vi "BU-SearchParamSpace.vi"(9 "Input String":string, 11 "UCF Param":string[][](table)) -> (2 "Req Param":string[](array[string]))   [LabVIEW 2014]
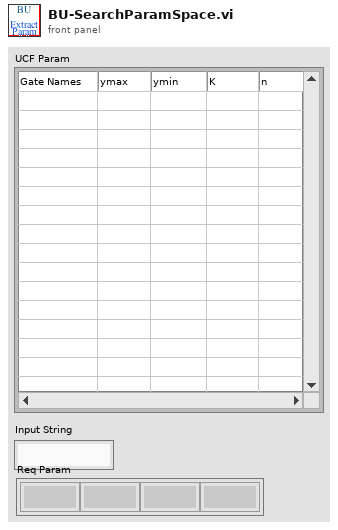
[diagram p1: front panel]
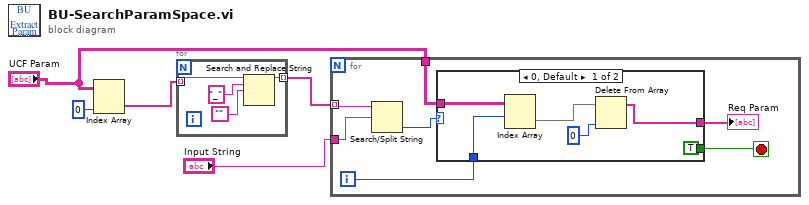
[diagram p0: block diagram]
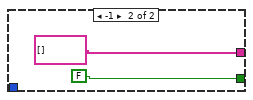
[diagram p2: hidden frame]
diagram:
  n1 = Index Array(array="UCF Param", index (col)=0 ("disabled index (col)")) -> (element=w2:string[])  [unwired: 1 in]
  n2 = for {
    tunnel: w2 -> [w7] mode=indexing
    tunnel: [w6] -> w1 mode=indexing
    n3 = Search and Replace String(input string=w7, search string="_", replace string="") -> (result string=w6:string)  [unwired: 5 in, 3 out]
  }
  n4 = for {
    tunnel: w1 -> [w16] mode=indexing
    tunnel: "Input String" -> [w15]
    tunnel: "UCF Param" -> [w13]
    i -> [w12]
    stop <- w11 stop-if-true
    n5 = Search/Split String(string=w16, search string/char (-)=w15) -> (offset of match=w14:i32)  [unwired: 1 in, 2 out]
    n6 = case shown="0, Default" w14 {
      tunnel: w13 -> [w22 _]
      tunnel: w12 -> [w21 _]
      tunnel: [TRUE FALSE] -> w11
      tunnel: [w17 string[] [] ("UCF Param")] -> w10
      frame 0, Default {
        n7 = Index Array(array=w22, index (row)=w21) -> (element=w19:string[])  [unwired: 1 in]
        n8 = Delete From Array(array=w19, index=0) -> (array with subset deleted=w17:string[])  [unwired: 1 in, 1 out]
      }
      frame -1 {
      }
    }
    "Req Param" <- w10
  }
